vi "IrInitialize.vi"(8 "error in (no error)":errorcluster) -> (0 "error out":errorcluster, 3 "Qbus out":refnum<class "Qbus.lvclass">)   [LabVIEW 2017]
uses:
  <vilib>/addons/Qbus/Qbus.lvclass
  <vilib>/addons/TraceLogger/TraceLogger.lvlib
  <vilib>/addons/SystemInfoProcess/SystemInfoProcess.lvlib
  <vilib>/addons/InsightCM/Utilities/GlobalConfiguration/GlobalConfiguration.lvlib
  <vilib>/addons/PointValueMap/PointValueMap.lvlib
  <vilib>/addons/cRIODetectHW/cRIODetectHW.lvlib
  <vilib>/addons/cRIODetectHW/control/cRIO Product Info.ctl
  <vilib>/addons/cRIODetectHW/control/SystemHW.ctl
  <vilib>/addons/PointValueMap/subVIs/Point_Write_variant.vi
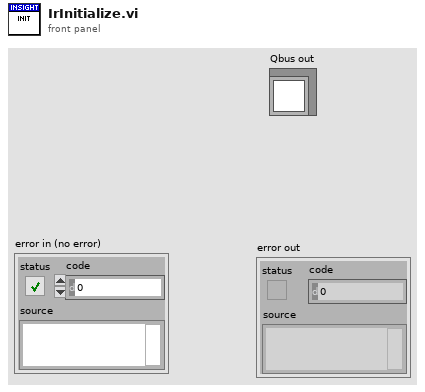
[diagram p1: front panel]
types:
  T1 = typedef "cRIODetectHW.lvlib/SystemHW.ctl" = cluster{"controller":T2, "chassis":T2, "modules":T2[]}
  T2 = typedef "cRIODetectHW.lvlib/cRIO Product Info.ctl" = cluster{"vendorName":string, "productName":string, "serialNumber":string}
  T3 = typedef "PointValueMap.lvlib/PointMap.ctl" = refnum<data-value>
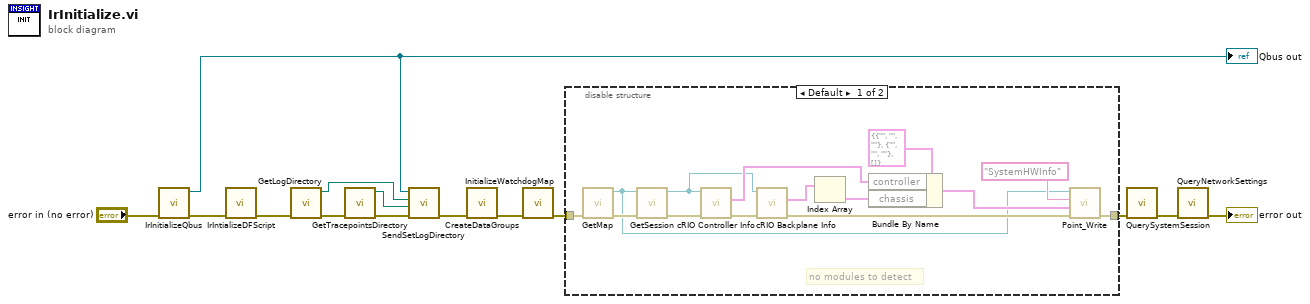
[diagram p0: block diagram]
diagram:
  n1 = call <vilib>:"IrInitializeQbus.vi"("error in (no error)"="error in (no error)") -> ("error out"=w11:errorcluster, "Qbus out"=w12:refnum<class "Qbus.lvclass">)  [unwired: 9 in]
  "Qbus out" <- w12
  n2 = call <vilib>:"IrIntializeDFScript.vi"("error in (no error)"=w11) -> ("error out"=w1:errorcluster)  [unwired: 10 in]
  n3 = call <vilib>:"GetLogDirectory.vi"("error in (no error)"=w1) -> ("error out"=w6:errorcluster, "log dir"=w8:path)  [unwired: 9 in]
  n4 = call <vilib>:"GetTracepointsDirectory.vi"("error in (no error)"=w6) -> ("error out"=w4:errorcluster, "application directory"=w5:path)  [unwired: 9 in]
  n5 = call <vilib>:"SendSetLogDirectory.vi"("error in (no error)"=w4, "tracpoint directory"=w5, "log directory"=w8, "qbus in"=w12) -> ("error out"=w13:errorcluster)  [unwired: 6 in, 1 out]
  n6 = call <vilib>:"CreateDataGroups.vi"("error in (no error)"=w13) -> ("error out"=w7:errorcluster)  [unwired: 10 in]
  n7 = call <vilib>:"InitializeWatchdogMap.vi"("error in (no error)"=w7) -> ("error out"=w3:errorcluster)  [unwired: 10 in]
  n8 = disable-structure shown="Default" {
    disable-tunnel: w3 -> [w26 _]
    disable-tunnel: [w17 _] -> w2
    frame condition #0 {
      # "no modules to detect"
      n9 = call <vilib>:"GetMap.vi"("error in (no error)"=w26) -> ("error out"=w27:errorcluster, "SystemInfoMap"=w16:T3)  [unwired: 9 in]
      n10 = call <vilib>:"GetSession.vi"("error in (no error)"=w27, "map"=w16) -> ("error out"=w22:errorcluster, "session"=w15:refnum<k21>)  [unwired: 8 in]
      n11 = call <vilib>:"cRIO Controller Info.vi"("error in (no error)"=w22, "session in"=w15) -> ("error out"=w25:errorcluster, "cRIO Controller Information"=w20:T2)  [unwired: 8 in]
      n12 = call <vilib>:"cRIO Backplane Info.vi"("error in (no error)"=w25, "session in"=w15) -> ("error out"=w18:errorcluster, "Chasses Info"=w24:T2[])  [unwired: 7 in, 1 out]
      n13 = Index Array(array=w24) -> (element=w21:T2)  [unwired: 1 in]
      n14 = Bundle By Name(cluster=T1 {"controller"={"vendorName"="", "productName"="", "serialNumber"=""}, "chassis"={"vendorName"="", "productName"="", "serialNumber"=""}, "modules"=[]} ("SystemHW"), "controller"=w20, "chassis"=w21) -> (w19:T1)
      n15 = call-poly <vilib>:"Point_Write.vi"("Error In"=w18, "Value"=w19, "Tag"="SystemHWInfo", "Map"=w16) -> ("Error Out"=w17:errorcluster)  [unwired: 6 in, 1 out]
    }
    frame condition #1 (active) {
    }
  }
  n16 = call <vilib>:"QuerySystemSession.vi"("error in (no error)"=w2) -> ("error out"=w10:errorcluster)  [unwired: 10 in]
  n17 = call <vilib>:"QueryNetworkSettings.vi"("error in (no error)"=w10) -> ("error out"=→"error out":errorcluster)  [unwired: 10 in]
